vi "test udp wr.vi"() -> ()   [LabVIEW 2019]
panel:
  out "포트":u16
  in  "dt":u32=50
  out "데이터 출력":string="2020-09-25 오후 7:56:47"
  in  "Stop":bool
  out "Current Data Value":dbl=0.4995100558362602
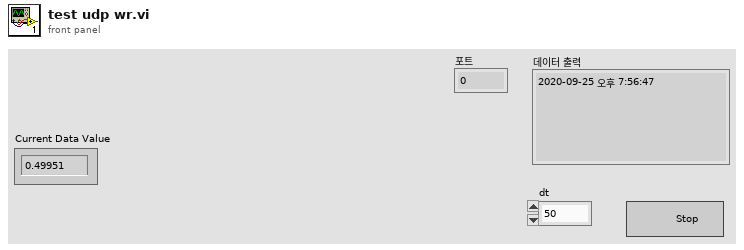
[diagram p1: front panel]
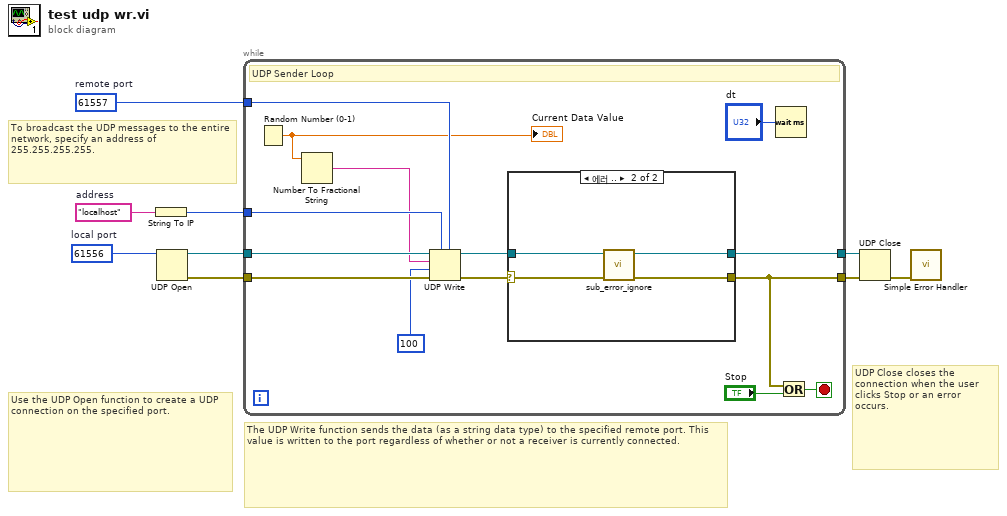
[diagram p0: block diagram]
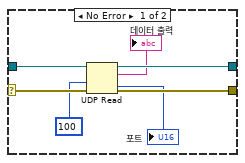
[diagram p2: hidden frame]
diagram:
  w1 = u16 61557  # remote port
  w2 = u16 61556  # local port
  w7 = "localhost"  # address
  # "To broadcast the UDP messages to the entire network, specify an address of 255.255.255.255."
  # "UDP Close closes the connection when the user clicks Stop or an error occurs."
  # "The UDP Write function sends the data (as a string data type) to the specified remote port. This value is written to the port regardless of whether or not a receiver is currently connected."
  # "Use the UDP Open function to create a UDP connection on the specified port."
  n1 = String To IP(1:w7) -> (0:w5:u32)
  n2 = UDP Open(11:w2) -> (port=w4:refnum<k16>, 0:w3:errorcluster)  [unwired: 4 in, 1 out]
  n3 = while {
    tunnel: [w13] -> w8
    tunnel: w4 -> [w23]
    tunnel: w3 -> [w22]
    tunnel: [w11] -> w9
    tunnel: w5 -> [w19]
    tunnel: w1 -> [w16]
    stop <- w21 stop-if-true
    # "UDP Sender Loop"
    n4 = Random Number (0-1)() -> (number: 0 to 1=w15:dbl)
    "Current Data Value" <- w15
    n5 = Number To Fractional String(number=w15) -> (F-format string=w17:string)  [unwired: 3 in]
    n6 = UDP Write(address=w19, port or service name=w16, connection ID=w23, data in=w17, 8:w22, 9:100 ("타임아웃 ms (25000)")) -> (error out=w14:errorcluster, 3:w12:refnum<k16>)
    n7 = case shown="에러 .." w14 {
      selector: w14 -> [w29 w32]
      tunnel: [w27 w31] -> w13
      tunnel: w12 -> [w30 w33]
      tunnel: [w28 w33] -> w11
      frame No Error {
        n8 = UDP Read(connection ID=w30, timeout ms (25000)=100 ("타임아웃 ms (25000)"), 8:w29) -> (data out=→"데이터 출력":string, error out=w27:errorcluster, 3:w28:refnum<k16>, 4:→"포트":u16)  [unwired: 1 in, 1 out]
      }
      frame Error {
        n9 = call "sub_error_ignore.vi"("error in"=w32) -> ("error out"=w31:errorcluster)  [unwired: 10 in]
      }
    }
    n10 = Wait (ms)(milliseconds to wait="dt") -> ()  [unwired: 1 out]
    n11 = Or(x=w13, y="Stop") -> (x .or. y?=w21:bool)
  }
  n12 = UDP Close(connection ID=w9, 8:w8) -> (error out=w6:errorcluster)  [unwired: 1 out]
  n13 = call <vilib>:"Simple Error Handler.vi"("error in (no error)"=w6) -> ()  [unwired: 4 in, 5 out]
